vi "Add Picture in Document.vi"(8 "error in (no error)":errorcluster, 10 "Picture Path":path, 11 "xwpfWriter in":refnum<class "xwpfWriter.lvclass">) -> (0 "error out":errorcluster, 3 "xwpfWriter out":refnum<class "xwpfWriter.lvclass">)   [LabVIEW 2017, in "xwpfWriter.lvclass"]
uses:
  xwpfWriter.lvclass
  xwpfWriter.lvclass/xwpfWriter.ctl
  C:/Users/Neo/Desktop/Dev_Tools_BR/LabVIEW_NPOI/src/lib/NPOI 2.1.1/NPOI.OOXML.dll
  lib/NPOI 2.1.1/NPOI.OOXML.dll
  Styles/Title/Title.lvclass
  C:/Users/Neo/Desktop/Dev_Tools_BR/LabVIEW_NPOI/src/Styles/Style/Style.lvclass
  Support/File Stream/File Stream.lvlib
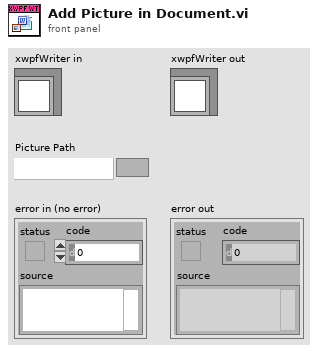
[diagram p1: front panel]
types:
  T1 = typedef "LabVIEW NPOI.lvlib/Picture Type.ctl" = i32
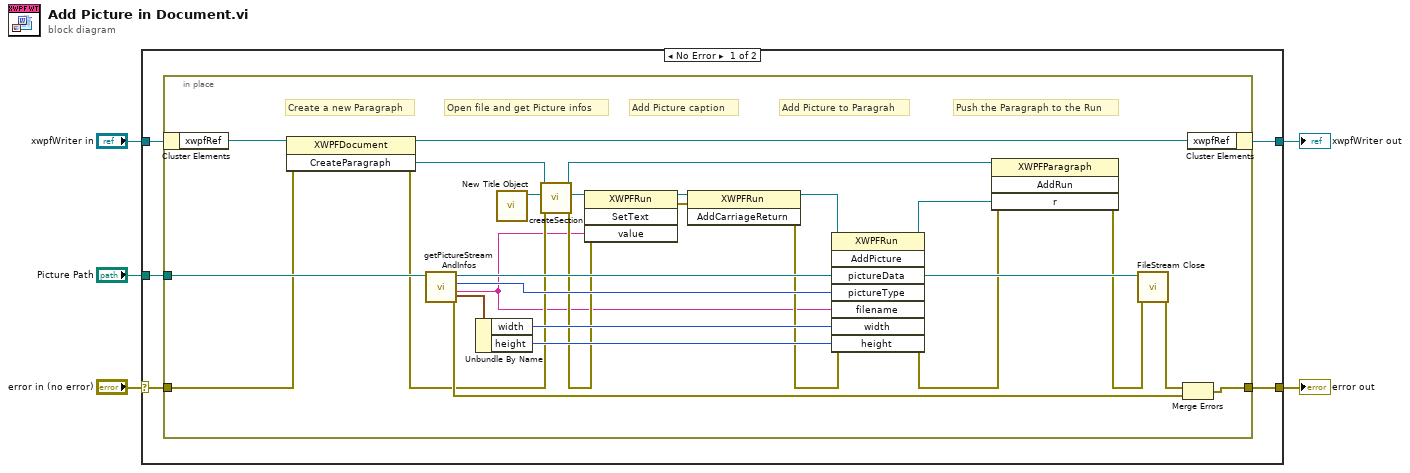
[diagram p0: block diagram]
diagram:
  n1 = case shown="No Error" "error in (no error)" {
    selector: "error in (no error)" -> [w9 w38]
    tunnel: [w8 w38] -> w4
    tunnel: [w6 w37] -> w2
    tunnel: "xwpfWriter in" -> [w10 w37]
    tunnel: "Picture Path" -> [w7 _]
    frame No Error {
      n2 = in-place {
        in-place-border: w7 -> [w33]
        in-place-border: [w35] -> w8
        in-place-border: w9 -> [w30]
        # "Push the Paragraph to the Run"
        # "Add Picture to Paragrah"
        # "Open file and get Picture infos"
        # "Add Picture caption"
        # "Create a new Paragraph"
        n3 = in-place-cluster #1(w10) -> ("xwpfRef"=w36:refnum<k24>)
        n4 = invoke class="XWPFDocument" method="CreateParagraph"(reference=w36, error in=w30) -> (reference out=w32:refnum<k24>, error out=w16:errorcluster, "CreateParagraph"=w14:refnum<k24>)  [unwired: 1 in]
        n5 = call "getPictureStreamAndInfos.vi"("Picture Path"=w33) -> ("error out"=w22:errorcluster, "File Name"=w12:string, "PictureType"=w29:T1, "FileStream out"=w31:refnum<k24>, "Picture Size"=w28:cluster{"width":i32, "height":i32})  [unwired: 6 in]
        n6 = Unbundle By Name(w28) -> ("width"=w27:i32, "height"=w26:i32)
        n7 = call "New Title Object.vi"() -> ("Title out"=w11:refnum<class "Title.lvclass">)  [unwired: 10 in, 1 out]
        n8 = call "createSection.vi"("error in (no error)"=w16, "Style"=w11, "Paragraph in"=w14) -> ("error out"=w18:errorcluster, "Section out"=w19:refnum<k24>, "Paragraph out"=w13:refnum<k24>)  [unwired: 6 in]
        n9 = invoke class="XWPFRun" method="SetText"(reference=w19, error in=w18, "value"=w12) -> (reference out=w20:refnum<k24>, error out=w21:errorcluster)  [unwired: 1 in, 2 out]
        n10 = invoke class="XWPFRun" method="AddCarriageReturn"(reference=w20, error in=w21) -> (reference out=w15:refnum<k24>, error out=w17:errorcluster)  [unwired: 1 in, 1 out]
        n11 = invoke class="XWPFRun" method="AddPicture"(reference=w15, error in=w17, "pictureData"=w31, "pictureType"=w29, "filename"=w12, "width"=w27, "height"=w26) -> (reference out=w25:refnum<k24>, error out=w24:errorcluster)  [unwired: 1 in, 6 out]
        n12 = invoke class="XWPFParagraph" method="AddRun"(reference=w13, error in=w24, "r"=w25) -> (error out=w23:errorcluster)  [unwired: 1 in, 3 out]
        n13 = call "FileStream Close.vi"("error in (no error)"=w23, "reference"=w31) -> ("error out"=w34:errorcluster)  [unwired: 9 in]
        n14 = Merge Errors(w34, w22) -> (w35:errorcluster)
        n15 = in-place-cluster #1("xwpfRef"=w32) -> (w6:refnum<class "xwpfWriter.lvclass">)
      }
    }
    frame Error {
    }
  }
  "error out" <- w4
  "xwpfWriter out" <- w2
